vi "MoveAbsolute.vi"(8 "error in (no error)":errorcluster, 10 "Move Abs Value":dbl, 11 "ThorlabsLabJack in":refnum<class "ThorlabsLabJack.lvclass">) -> (0 "error out":errorcluster, 3 "ThorlabsLabJack out":refnum<class "ThorlabsLabJack.lvclass">)   [LabVIEW 2018, in "ThorlabsLabJack.lvlib" / "ThorlabsLabJack.lvclass"]
uses:
  ThorlabsLabJack.lvclass
  ThorlabsLabJack.lvclass/ThorlabsLabJack.ctl
  C:/Projects/LabVIEW/In-Progress/Chetan Malpure/Axis/Thorlabs LabJack/Drivers/Thorlabs.MotionControl.IntegratedStepperMotorsCLI.dll
  Drivers/Thorlabs.MotionControl.IntegratedStepperMotorsCLI.dll
  91b5fc19-c8fb-4e29-ae9f-d63fcf16b306.vi
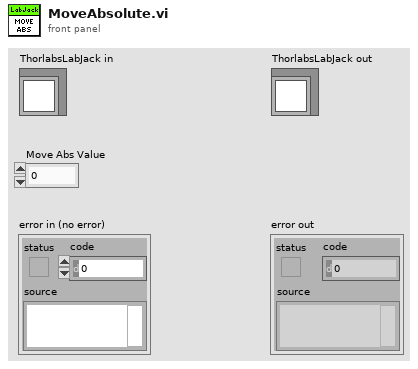
[diagram p1: front panel]
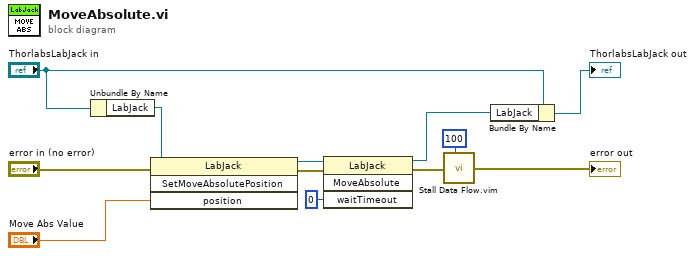
[diagram p0: block diagram]
diagram:
  n1 = Unbundle By Name("ThorlabsLabJack in") -> ("LabJack"=w4:refnum<k24>)
  n2 = invoke class="LabJack" method="SetMoveAbsolutePosition"(reference=w4, error in="error in (no error)", "position"="Move Abs Value") -> (reference out=w2:refnum<k24>, error out=w5:errorcluster)  [unwired: 1 in, 2 out]
  n3 = invoke class="LabJack" method="MoveAbsolute"(reference=w2, error in=w5, "waitTimeout"=0) -> (reference out=w6:refnum<k24>, error out=w7:errorcluster)  [unwired: 1 in, 2 out]
  n4 = call "Stall Data Flow.vim"("value in"=w7, "milliseconds to wait"=u32 100) -> ("value out"=→"error out":errorcluster)  [unwired: 1 out]
  n5 = Bundle By Name(cluster="ThorlabsLabJack in", "LabJack"=w6) -> (→"ThorlabsLabJack out":refnum<class "ThorlabsLabJack.lvclass">)
